vi "output-wavelength.vi"(2 "set pixel width":sgl, 3 "Set Number Pixels":u32) -> (1 "wavelength array":sgl[](array[numeric]), 6 "Set Pixel Width":u32, 7 "Set Number Pixels":u32, 9 "Wavelength Last Pixel":sgl, 10 "Wavelength First Pixel":sgl)   [LabVIEW 2017]
uses:
  ShamrockCIF.dll
panel:
  in  "error in (no error)":errorcluster
  out "error out":errorcluster
  out "SHAMROCK_COMMUNICATION_ERROR":i32
  out "SHAMROCK_NOT_INITIALIZED":i32
  # "CALIBRATION"
  # "ACTIONS"
  # "SDK RETURN VALUES"
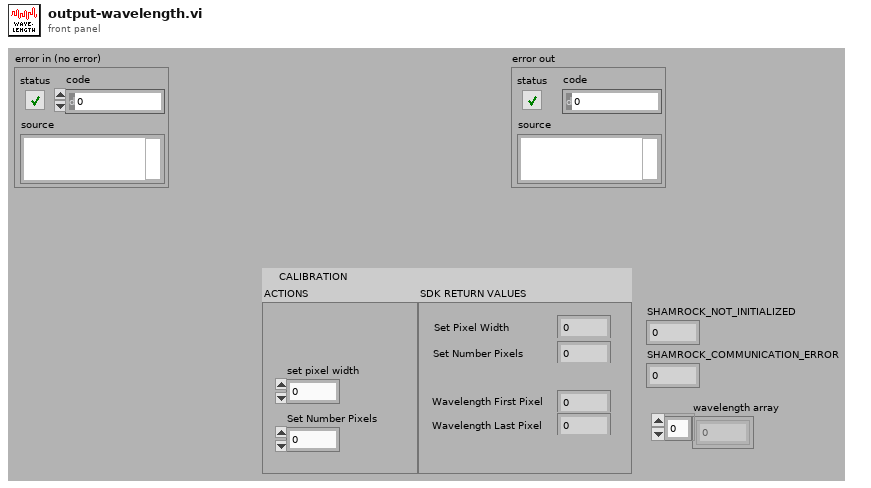
[diagram p1: front panel]
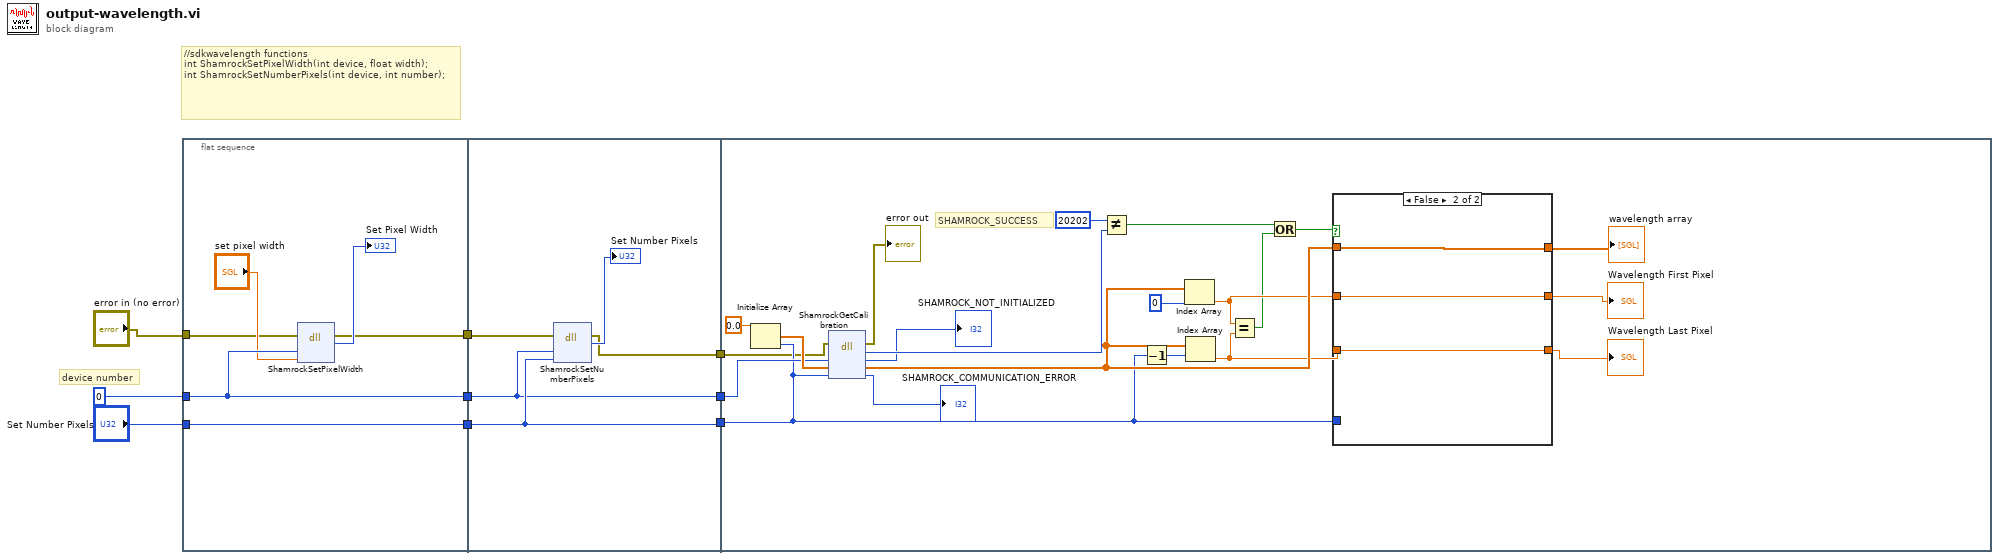
[diagram p0: block diagram]
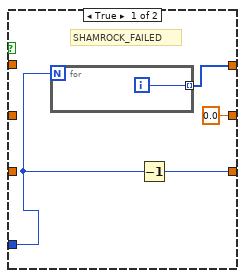
[diagram p2: hidden frame]
diagram:
  # "device number"
  # "//sdkwavelength functions\nint ShamrockSetPixelWidth(int device, float width);\nint ShamrockSetNumberPixels(int device, int number);"
  n1 = flat-sequence {
    tunnel: 0 ("Device No") -> [w14]
    tunnel: [w14] -> w8
    tunnel: "Set Number Pixels" -> [w13]
    tunnel: [w13] -> w6
    tunnel: [w12] -> w5
    tunnel: "error in (no error)" -> [w10]
    tunnel: w8 -> [w17]
    tunnel: w6 -> [w18]
    tunnel: w5 -> [w19]
    tunnel: [w18] -> w4
    tunnel: [w17] -> w3
    tunnel: [w16] -> w2
    tunnel: w4 -> [w23]
    tunnel: w3 -> [w24]
    tunnel: w2 -> [w22]
    frame #0 {
      n2 = dll-call lib="ShamrockCIF.dll" fn="ShamrockSetPixelWidth"(error in=w10, w14, "set pixel width") -> (error out=w12:errorcluster, →"Set Pixel Width":i32)  [unwired: 4 in, 1 out]
    }
    frame #1 {
      n3 = dll-call lib="ShamrockCIF.dll" fn="ShamrockSetNumberPixels"(error in=w19, w17, w18) -> (error out=w16:errorcluster, →"Set Number Pixels":i32)  [unwired: 4 in, 1 out]
    }
    frame #2 {
      # "SHAMROCK_SUCCESS"
      n4 = Initialize Array(sgl 0.0, w23) -> (w25:sgl[])
      n5 = dll-call lib="ShamrockCIF.dll" fn="ShamrockGetCalibration"(error in=w22, w24, w25, w23) -> (error out=→"error out":errorcluster, w31:i32, →"SHAMROCK_NOT_INITIALIZED":i32, w41:sgl[], →"SHAMROCK_COMMUNICATION_ERROR":i32)  [unwired: 2 in, 1 out]
      n6 = Not Equal?(x=20202, y=w31) -> (x != y?=w33:bool)
      n7 = Decrement(x=w23) -> (x-1=w30:u32)
      n8 = Index Array(array=w41, index=0) -> (element=w37:sgl)
      n9 = Index Array(array=w41, index=w30) -> (element=w39:sgl)
      n10 = Equal?(x=w37, y=w39) -> (x = y?=w34:bool)
      n11 = Or(x=w33, y=w34) -> (x .or. y?=w35:bool)
      n12 = case shown="False" w35 {
        tunnel: [sgl 0.0 w48] -> w38
        tunnel: [w43 w49] -> w40
        tunnel: [w44 w47] -> w36
        tunnel: w37 -> [_ w48]
        tunnel: w39 -> [_ w49]
        tunnel: w41 -> [_ w47]
        tunnel: w23 -> [w42 _]
        frame True {
          # "SHAMROCK_FAILED"
          n13 = for {
            N: w42 -> [_]
            tunnel: [w46] -> w44 mode=indexing
            i -> [w46]
          }
          n14 = Decrement(x=w42) -> (x-1=w43:u32)
        }
        frame False {
        }
      }
      "Wavelength First Pixel" <- w38
      "Wavelength Last Pixel" <- w40
      "wavelength array" <- w36
    }
  }
